vi "Write Blue DAQ.vi"(8 "error in (no error)":errorcluster, 10 "Blue DAQ":T1={"Rate (MHz)"=4.0, "Laser Rep (Hz)"=2000.0, "Laser DC (%)"=0.5}, 11 "eCRDS in":refnum<class "eCRDS.lvclass">) -> (0 "error out":errorcluster, 3 "eCRDS out":refnum<class "eCRDS.lvclass">)   [LabVIEW 2014, in "eCRDS Library.lvlib" / "eCRDS.lvclass"]
uses:
  eCRDS.lvclass
  eCRDS.lvclass/eCRDS.ctl
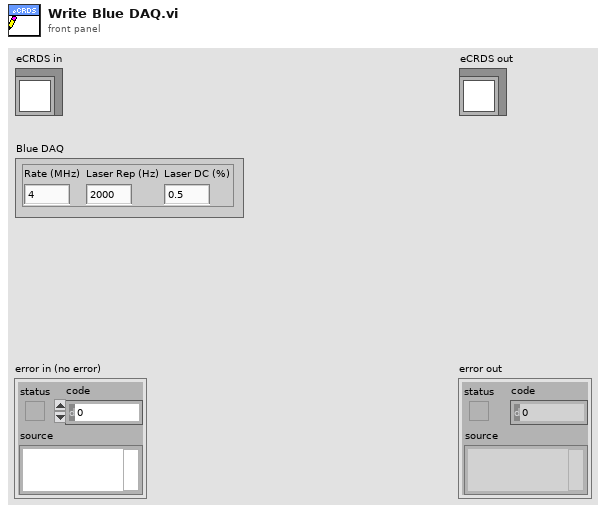
[diagram p1: front panel]
types:
  T1 = cluster{"Rate (MHz)":dbl, "Laser Rep (Hz)":dbl, "Laser DC (%)":dbl}
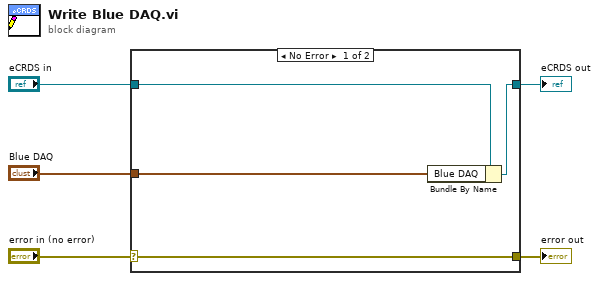
[diagram p0: block diagram]
diagram:
  n1 = case shown="No Error" "error in (no error)" {
    selector: "error in (no error)" -> [w9 w10]
    tunnel: [w9 w10] -> w4
    tunnel: [w7 w11] -> w2
    tunnel: "eCRDS in" -> [w8 w11]
    tunnel: "Blue DAQ" -> [w6 _]
    frame No Error {
      n2 = Bundle By Name(cluster=w8, "Blue DAQ"=w6) -> (w7:refnum<class "eCRDS.lvclass">)
    }
    frame Error {
    }
  }
  "error out" <- w4
  "eCRDS out" <- w2
